vi "DFD Save NStage MRate Filter to Text File.vi"(8 "error in (no error)":errorcluster, 9 "comments":string, 10 "file path in":path, 11 "multirate filters in":T1[](array[typedef]) {"mMRate_SumWl" min=1 max=32 step=1; "mMRate_InputIwl" min=1 max=32 step=1; "mMRate_GainWl" min=1 max=32 step=1; "mMRate_OutputWl" min=1 max=32 step=1; "mMRate_InputWl" min=1 max=32 step=1; "mMRate_CoefWl" min=1 max=32 step=1; "mMRate_Mode" items=["Default"=-1, "No Rate Change"=0, "Interpolation"=1, "Decimation"=2, "Interpolated"=3, "Rational"=4]}) -> (0 "error out":errorcluster, 2 "file path out":path, 3 "multirate filters out":T1[](array[typedef]) {"mMRate_SumWl" min=1 max=32 step=1; "mMRate_InputIwl" min=1 max=32 step=1; "mMRate_GainWl" min=1 max=32 step=1; "mMRate_OutputWl" min=1 max=32 step=1; "mMRate_InputWl" min=1 max=32 step=1; "mMRate_CoefWl" min=1 max=32 step=1; "mMRate_Mode" items=["Default"=-1, "No Rate Change"=0, "Interpolation"=1, "Decimation"=2, "Interpolated"=3, "Rational"=4]})   [LabVIEW 2017, in "NI_DigFilterLicensed.lvlib"]
doc: "Saves a filter or a filter bank to a text file in XML format. Wire data to the <B>filter in</B> input to determine the polymorphic instance to use or manually select the instance."
uses:
  <vilib>/addons/Digital Filter Design/NI_DigFilterLicensed.lvlib
  <vilib>/addons/Digital Filter Design/_Objects.llb/DFD Multirate Filter Obj.ctl
  <vilib>/addons/Digital Filter Design/_Objects.llb/DFD Multirate Mode.ctl
  <vilib>/addons/Digital Filter Design/_Objects.llb/DFD Coef Norm Type.ctl
  <vilib>/addons/Digital Filter Design/_Objects.llb/DFD Round-off Mode.ctl
  <vilib>/addons/Digital Filter Design/_Objects.llb/DFD FXP MRate Multiply Mode.ctl
  <vilib>/addons/Digital Filter Design/_Misc.llb/dfd_Error Handlers (Single).vi
  <vilib>/addons/Digital Filter Design/NI_DigFilter_Process.lvlib
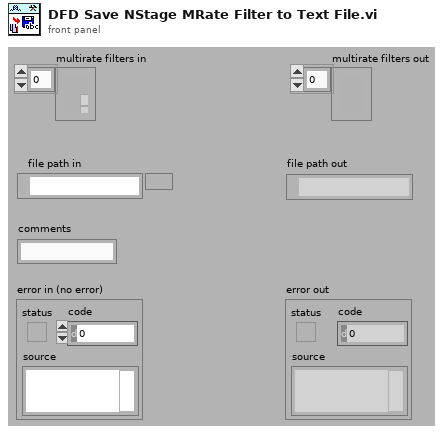
[diagram p1: front panel]
types:
  T1 = typedef "NI_DigFilterLicensed.lvlib/DFD Multirate Filter Obj.ctl" = cluster{"mMRate_Structure":enum16{"CIC", "FIR", "IIR", "Lattice"}, "mMRate_Mode":T2, "mMRate_Factor":i32, "mMRate_FIRParams":cluster{"mMRate_FIR_H":dbl[], "mMRate_FIR_IsNyquist?":bool, "mMRate_FIR_IsSymmetric?":bool}, "mMRate_CICParams":cluster{"mMRate_CIC_#Stage":i32, "mMRate_CIC_Lag":i32, "mMRate_CIC_Type":enum16{"Lowpass", "Highpass"}}, "mMRate_Order":i32, "mMRate_Version":string, "mMRate_Comments":string, "mMRate_RationalFactor":cluster{"mMRate_L":i32, "mMRate_M":i32}, "mMRate_Fs":dbl, "mMRate_Quantized?":bool, "mMRate_QFilterGain":dbl, "mMRate_CoefWl":i16, "mMRate_Scaling":cluster{"mMRate_ScaleByPowerOf2?":bool, "mMRate_ScaleType":T3}, "mMRate_InputWl":i16, "mMRate_OutputWl":i16, "mMRate_OutputMode":T4, "mMRate_MultMode":T5, "mMRate_BitPruning":bool, "mMRate_GainWl":i16, "mMRate_OutputFwl":i16, "mMRate_SumIwl":i16, "mMRate_InputIwl ":i16, "mMRate_SumWl":i16, "mMRate_CoefIwl":i16}
  T2 = typedef "NI_DigFilterLicensed.lvlib/DFD Multirate Mode.ctl" = i16
  T3 = typedef "NI_DigFilterLicensed.lvlib/DFD Coef Norm Type.ctl" = enum16{"No Norm", "Time Domain 1-Norm", "Time Domain 2-Norm", "Time Domain Inf-Norm"}
  T4 = typedef "NI_DigFilterLicensed.lvlib/DFD Round-off Mode.ctl" = enum16{"Nearest", "Truncation"}
  T5 = typedef "NI_DigFilterLicensed.lvlib/DFD FXP MRate Multiply Mode.ctl" = enum16{"Truncated", "Full"}
  T6 = enum16{"open", "open or create", "create or replace", "create", "open (read only)"}
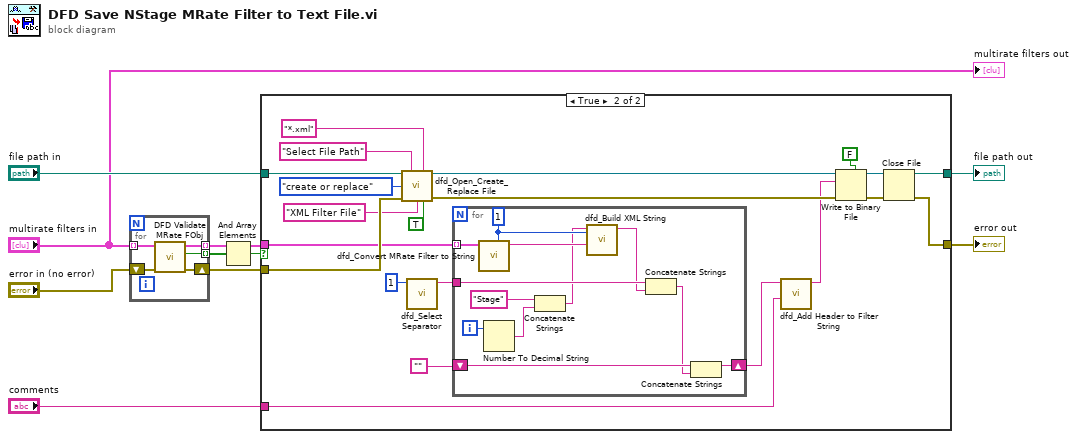
[diagram p0: block diagram]
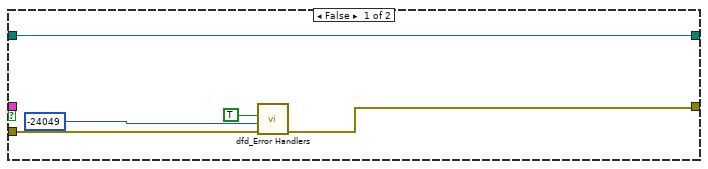
[diagram p2: hidden frame]
diagram:
  n1 = for {
    tunnel: [w15] -> w6 mode=indexing
    tunnel: [w13] -> w4 mode=indexing
    shift-right: [w12] -> w3
    shift-left: "error in (no error)" -> [w14]
    tunnel: "multirate filters in" -> [w11] mode=indexing
    n2 = call <vilib>:"DFD Validate MRate FObj.vi"("error in (no error)"=w14, "multirate filter in"=w11) -> ("error out"=w12:errorcluster, "is valid FLP?"=w13:bool, "multirate filter out"=w15:T1)  [unwired: 7 out]
  }
  n3 = And Array Elements(Boolean array=w4) -> (logical AND=w2:bool)
  n4 = case shown="True" w2 {
    tunnel: [w16 w37] -> w10
    tunnel: [w20 w33] -> w9
    tunnel: "file path in" -> [w20 w41]
    tunnel: "comments" -> [_ w29]
    tunnel: w6 -> [_ w25]
    tunnel: w3 -> [w19 w27]
    frame False {
      n5 = call-poly <vilib>:"dfd_Error Handlers.vi"("error in (no error)"=w19, "error code"=-24049 ("ERR_INVALID_MULTIRATE_FILTER"), "condition failed?"=TRUE) -> ("error out"=w16:errorcluster)  [unwired: 8 out]
    }
    frame True {
      n6 = call <vilib>:"dfd_Open_Create_Replace File.vi"("file path"=w41, "prompt"="Select File Path" ("Prompt"), "pattern"="*.xml", "function (open:0)"=T6."create or replace", "error in (no error)"=w27, "pattern label"="XML Filter File" ("Prompt"), "advisory dialog? (display:T)"=TRUE) -> ("refnum"=w36:refnum<file>, "error out"=w39:errorcluster)  [unwired: 2 in, 5 out]
      n7 = call <vilib>:"dfd_Select Separator.vi"("indent order"=1) -> ("separator"=w24:string)  [unwired: 10 out]
      n8 = for {
        tunnel: w25 -> [w53] mode=indexing
        tunnel: w24 -> [w52]
        shift-right: [w43] -> w21
        shift-left: "" -> [w44]
        i -> [w51]
        w50 = 1 ("indent order")
        n9 = call <vilib>:"dfd_Convert MRate Filter to String.vi"("indent order"=w50, "multirate filter in"=w53) -> ("xml string"=w48:string)  [unwired: 1 in, 8 out]
        n10 = Number To Decimal String(number=w51) -> (decimal integer string=w46:string)  [unwired: 1 out]
        n11 = Concatenate Strings("Stage" ("string"), w46) -> (w45:string)
        n12 = call <vilib>:"dfd_Build XML String.vi"("indent order"=w50, "string in"=w48, "element name"=w45) -> ("xml string out"=w49:string)  [unwired: 1 in, 7 out]
        n13 = Concatenate Strings(w52, w49) -> (w42:string)
        n14 = Concatenate Strings(w44, w42) -> (w43:string)
      }
      n15 = call <vilib>:"dfd_Add Header to Filter String.vi"("customer comments"=w29, "string in"=w21) -> ("string out"=w28:string)  [unwired: 9 out]
      n16 = Write to Binary File(file (use dialog)=w36, data=w28, error in=w39, 5:FALSE ("prepend array or string size? (T)")) -> (refnum out=w34:refnum<file>, error out=w38:errorcluster)  [unwired: 3 out]
      n17 = Close File(refnum=w34, error in=w38) -> (path=w33:path, error out=w37:errorcluster)
    }
  }
  "error out" <- w10
  "file path out" <- w9
  "multirate filters out" <- "multirate filters in"
